vi "New Terminal Enabled State Binding.vi"(7 "Initial State (T)":bool=TRUE, 8 "FALSE State (Disabled and Grayed Out)":T1(ring), 9 "TRUE State (Enabled)":T1(ring), 10 "Control":refnum<vi>) -> (0 "error out":errorcluster, 3 "TerminalEnabledStateBinding Out":refnum<class "TerminalEnabledStateBinding.lvclass">)   [LabVIEW 2017, in "Transport.lvlib" / "TerminalEnabledStateBinding.lvclass"]
doc: "<License>\nCopyright © 2017 Composed Systems, LLC | All rights reserved\nwww.composed.io\n\nAuthor: Ethan Stern <ethan.stern@composed.io>\n\nThis software is provided \"AS IS\" WITHOUT WARRANTIES, either express or implied, AND IS FOR EDUCATIONAL PURPOSES ONLY.\n</License>"
uses:
  TerminalEnabledStateBinding.lvclass
  TerminalEnabledStateBinding.lvclass/TerminalEnabledStateBinding.ctl
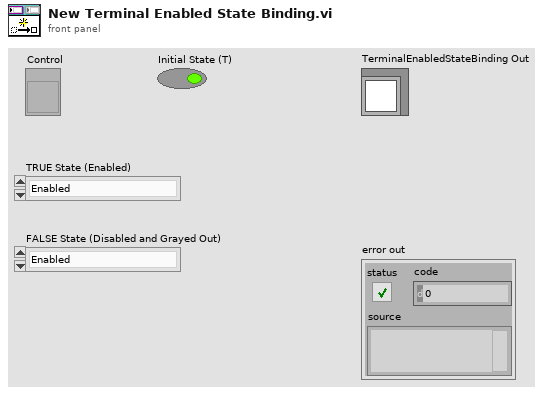
[diagram p1: front panel]
types:
  T1 = enum8{"Enabled", "Disabled", "Disabled and Grayed Out"}
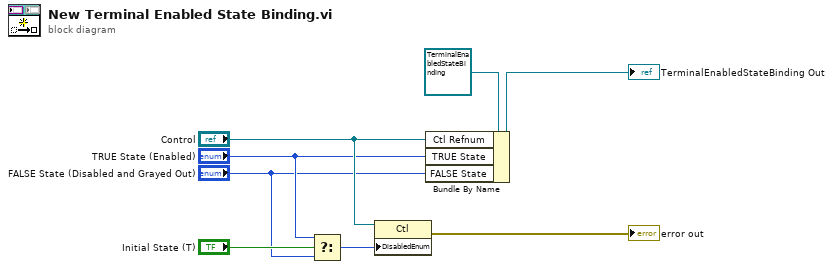
[diagram p0: block diagram]
diagram:
  n1 = Select(t="TRUE State (Enabled)", s="Initial State (T)", f="FALSE State (Disabled and Grayed Out)") -> (s? t:f=w1:T1)
  n2 = property class="Ctl"(reference="Control", "DisabledEnum"=w1) -> (error out=→"error out":errorcluster)  [unwired: 1 in, 1 out]
  n3 = Bundle By Name(cluster=refnum<class "TerminalEnabledStateBinding.lvclass"> refnum ("TerminalReference in"), "Ctl Refnum"="Control", "TRUE State"="TRUE State (Enabled)", "FALSE State"="FALSE State (Disabled and Grayed Out)") -> (→"TerminalEnabledStateBinding Out":refnum<class "TerminalEnabledStateBinding.lvclass">)
